vi "LuaVIEW Push (nil).vi"(5 "LuaVIEW reference in":T1, 11 "error in (no error)":errorcluster) -> (6 "LuaVIEW reference out":T1, 15 "error out":errorcluster)   [LabVIEW 2013]
doc: "Pushes a nil data item onto the Lua stack. This VI is part of a polymorphic set that supports various data types. To change the type being pushed, pop up on this VI's diagram icon and use the \"Select Type\" sub menu. When \"automatic\" is checked in that menu, wiring a different type to the top left input will cause the appropriate VI to be selected automatically."
uses:
  typedefs/t_LuaVIEW Reference.ctl
  typedefs/et_LuaVIEW CIN Actions.ctl
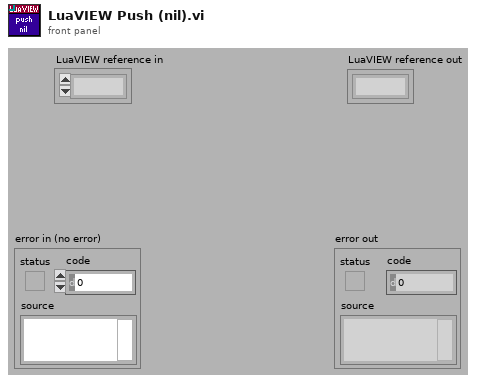
[diagram p1: front panel]
types:
  T1 = typedef "t_LuaVIEW Reference.ctl" = refnum<k1>
  T2 = typedef "et_LuaVIEW CIN Actions.ctl" = enum16{"checksynopsis", "_open", "_registerpublic", "_registerexport", "__never_an_error_result_ns", "luaversion", "cinversion", "_totals", "_taskcount", "pathological", "_unregnextpublic", "registryusecount", "__per_state_actions", "regsetprivate", "regsetindex", "regsetmodule", "_revokeexports", "_usepublic", "prepare", "compile", "execute", "call", "unregstaterefs", "_close", "pullboolean", "pullnumber", "pullI8", "pullU8", "pullI16", "pullU16", "pullI32", "pullU32", "pullobject", "pullrefnum", "pullstring", "pullflat", "pushflat", "pushobject", "getattribute", "setattribute", "stacktostring", "_startyieldtest", "_endyieldtest", "_pollprintbuffer", "__never_an_error_result_ps", "_pollexport", "setclone", "forcecleanup", "gettop", "clearstack", "insert", "pushboolean", "pushnumber", "pushrefnum", "pushstring", "pushnil", "pushvalue", "gettaskref", "settaskref"}
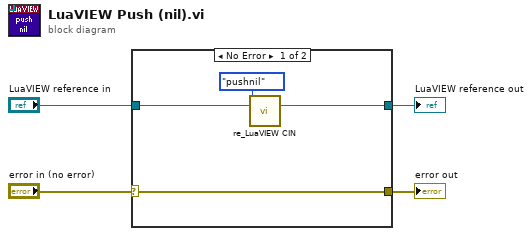
[diagram p0: block diagram]
diagram:
  n1 = case shown="No Error" "error in (no error)" {
    selector: "error in (no error)" -> [w6 w10]
    tunnel: [w5 w9] -> w4
    tunnel: [w6 w10] -> w3
    tunnel: "LuaVIEW reference in" -> [w7 w9]
    frame No Error {
      n2 = call "re_LuaVIEW CIN.vi"("action"=et_LuaVIEW_CIN_Actions."pushnil", "LuaVIEW reference in"=w7) -> ("LuaVIEW reference out"=w5:T1)  [unwired: 7 in, 6 out]
    }
    frame Error {
    }
  }
  "LuaVIEW reference out" <- w4
  "error out" <- w3
